vi "subItemThird.vi"(6 "single frequency":string, 7 "single frequency value":string, 8 "single frequency result":string, 9 "SN":string, 10 "third test item name":string, 11 "subIDcount":i32) -> (2 "SubItem":string)   [LabVIEW 2011]
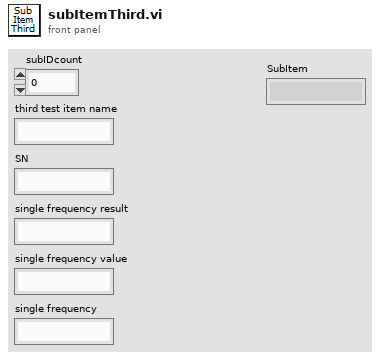
[diagram p1: front panel]
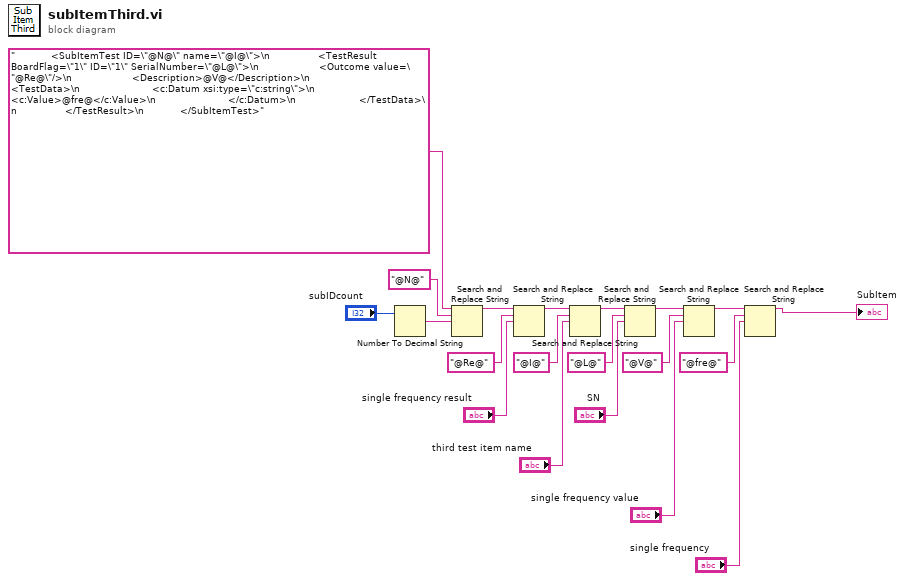
[diagram p0: block diagram]
diagram:
  n1 = Number To Decimal String(number="subIDcount") -> (decimal integer string=w18:string)  [unwired: 1 in]
  n2 = Search and Replace String(input string="            <SubItemTest ID=\"@N@\" name=\"@I@\">\n                <TestResult BoardFlag=\"1\" ID=\"1\" SerialNumber=\"@L@\">\n                    <Outcome value=\"@Re@\"/>\n                    <Description>@V@</Description>\n                    <TestData>\n                        <c:Datum xsi:type=\"c:string\">\n                            <c:Value>@fre@</c:Value>\n                        </c:Datum>\n                     </TestData>\n                </TestResult>\n            </SubItemTest>", search string="@N@" ("搜索字符串"), replace string=w18) -> (result string=w10:string)  [unwired: 5 in, 3 out]
  n3 = Search and Replace String(input string=w10, search string="@Re@" ("搜索字符串"), replace string="single frequency result") -> (result string=w8:string)  [unwired: 5 in, 3 out]
  n4 = Search and Replace String(input string=w8, search string="@I@" ("搜索字符串"), replace string="third test item name") -> (result string=w16:string)  [unwired: 5 in, 3 out]
  n5 = Search and Replace String(input string=w16, search string="@L@" ("搜索字符串"), replace string="SN") -> (result string=w13:string)  [unwired: 5 in, 3 out]
  n6 = Search and Replace String(input string=w13, search string="@V@" ("搜索字符串"), replace string="single frequency value") -> (result string=w12:string)  [unwired: 5 in, 3 out]
  n7 = Search and Replace String(input string=w12, search string="@fre@" ("搜索字符串"), replace string="single frequency") -> (result string=→"SubItem":string)  [unwired: 5 in, 3 out]
